vi "VSSNavigation.vi"(0 "output angle":dbl, 4 "output xy":dbl, 6 "Debug":bool, 8 "GoTo Navigation":bool, 11 "IA State Output in":T1) -> (3 "IA State Output out":T1)   [LabVIEW 2018]
uses:
  Vision_class/Old vision/SSL Detection Frame Simple Estimator Cameras VelCmd Folder/Core/AI Input.ctl
  Vision_class/Old vision/Controls/AI Robot.ctl
  Vision_class/Old vision/Controls/Functions Enum.ctl
  Vision_class/Old vision/Controls/AttackerStates.ctl
  Vision_class/Old vision/Controls/PathDests.ctl
  Vision_class/Old vision/Controls/PathDest.ctl
  VSSAttackerStates.ctl
  Vision_class/Old vision/SSL Detection Frame Simple Estimator Cameras VelCmd Folder/Core/AI Ball.ctl
  Vision_class/Old vision/SSL Detection Frame Simple Estimator Cameras VelCmd Folder/Core/Field Size.ctl
  Vision_class/Old vision/SSL Detection Frame Simple Estimator Cameras VelCmd Folder/Core/AI Judge.ctl
  Communication_class/Paths/MessageAI_State Folder/Intel/Command Enum.ctl
  Vision_class/Old vision/SSL Detection Frame Simple Estimator Cameras VelCmd Folder/Util/Events/Events.ctl
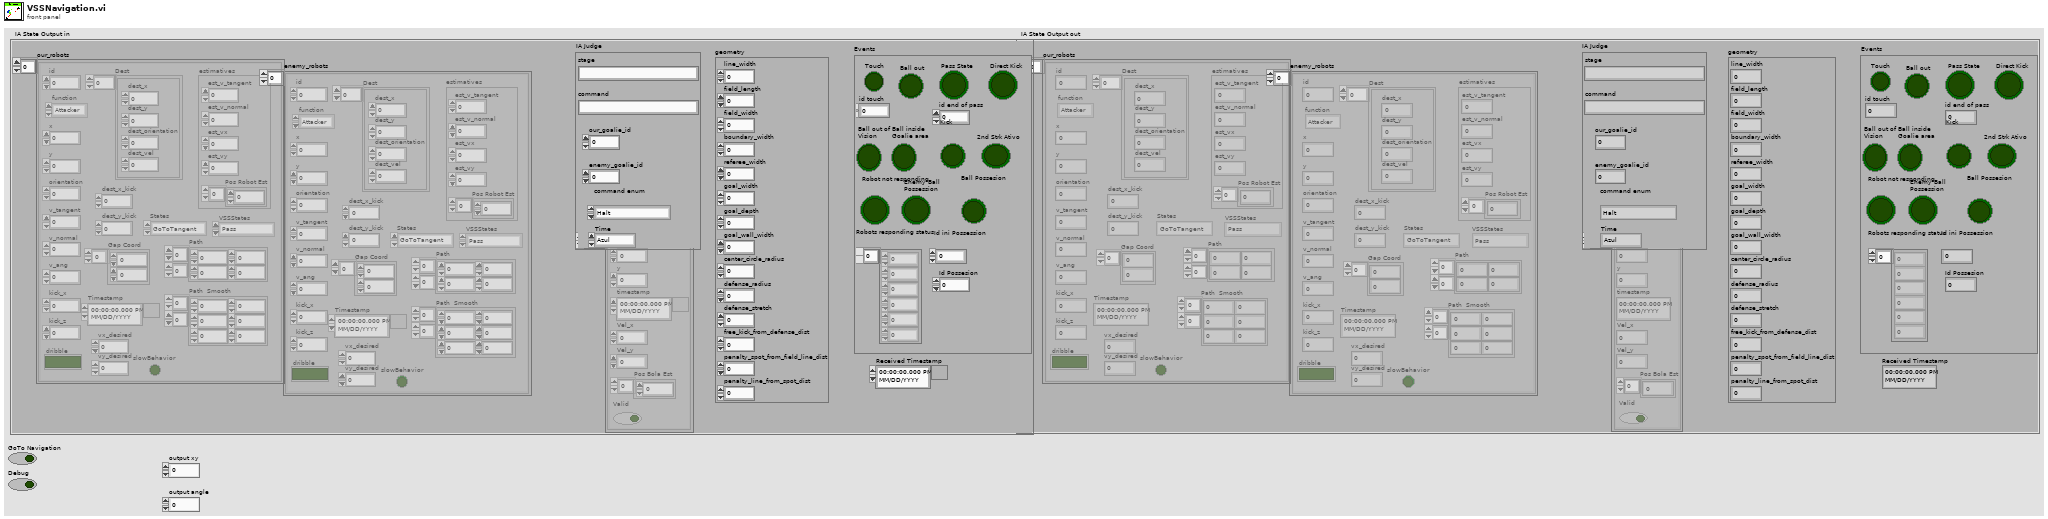
[diagram p1: front panel]
types:
  T1 = typedef "AI Input.ctl" = cluster{"our_robots":T2[], "enemy_robots":T2[], "balls":T8[], "geometry":T9, "IA Judge":T10, "Received Timestamp":timestamp, "Events":T12}
  T2 = typedef "AI Robot.ctl" = cluster{"id":u32, "function":T3, "x":dbl, "y":dbl, "orientation":dbl, "v_tangent":dbl, "v_normal":dbl, "v_ang":dbl, "kick_x":dbl, "kick_z":dbl, "dribble":bool, "Timestamp":timestamp, "estimatives":cluster{"est_v_tangent":dbl, "est_v_normal":dbl, "est_vx":dbl, "est_vy":dbl, "Pos Robot Est":dbl[]}, "dest_x_kick":dbl, "dest_y_kick":dbl, "Gap Coord":dbl[], "States":T4, "Path ":dbl[][], "Path  Smooth":dbl[][], "Dest":T5, "vx_desired":dbl, "vy_desired":dbl, "slowBehavior":bool, "VSSStates":T7}
  T3 = typedef "Functions Enum.ctl" = enum16{"2nd Striker", "Attacker", "Goalie", "Defender", "Striker", "Goto 0", "Dummy", "Kicker", "ZigZag 0", "ZigZag 1", "ZigZag 2", "ZigZag 3", "ZigZag 4", "ZigZag 5", "ZigZag 6", "ZigZag 7", "ZigZag 8", ""}
  T4 = typedef "AttackerStates.ctl" = enum16{"Pass", "GoToTangent", "BallGetting", "GoToKick", ""}
  T5 = typedef "PathDests.ctl" = T6[]
  T6 = typedef "PathDest.ctl" = cluster{"dest_x":dbl, "dest_y":dbl, "dest_orientation":dbl, "dest_vel":dbl}
  T7 = typedef "VSSAttackerStates.ctl" = enum16{"Pass", "GoToTangent", "BallGetting", "GoToKick", "Rotate anti-clockwise", "Rotate Clockwise", ""}
  T8 = typedef "AI Ball.ctl" = cluster{"x":dbl, "y":dbl, "timestamp":timestamp, "Vel_x":dbl, "Vel_y":dbl, "Pos Bola Est":dbl[], "Valid":bool}
  T9 = typedef "Field Size.ctl" = cluster{"line_width":u32, "field_length":u32, "field_width":u32, "boundary_width":u32, "referee_width":u32, "goal_width":u32, "goal_depth":u32, "goal_wall_width":u32, "center_circle_radius":u32, "defense_radius":u32, "defense_stretch":u32, "free_kick_from_defense_dist":u32, "penalty_spot_from_field_line_dist":u32, "penalty_line_from_spot_dist":u32}
  T10 = typedef "AI Judge.ctl" = cluster{"stage":string, "command":string, "our_goalie_id":dbl, "enemy_goalie_id":dbl, "command enum":T11, "Time":enum16{"Azul", "Amarelo"}}
  T11 = typedef "Command Enum.ctl" = enum16{"Halt", "Stop", "Force Start", "PKA Normal Start", "Prepare Kickoff Ally", "PKE Normal Start", "Prepare Kickoff Enemy", "Prepare Penalty Ally", "PPA Normal Start", "Prepare Penalty Enemy", "PPE Normal Start", "Direct Free Enemy", "Direct Free Ally", "Indirect Free Enemy", "Indirect Free Ally", "Timeout Enemy", "Timeout Ally", "Goal Enemy", "Goal Ally", "Ball Placement Enemy", "Ball Placement Ally", "Normal Half Time", "Extra Time Break", "Extra Half Time", "None", "Post Game"}
  T12 = typedef "Events.ctl" = cluster{"Touch":bool, "Ball out":bool, "id touch":dbl, "Ball out of \nVision":bool, "Ball inside \nGoalie area":bool, "Robot not responding":bool, "Robots responding status":dbl[], "Enemy Ball \nPossession":bool, "Pass State":bool, "id end of pass":dbl, "Kick":bool, "Id ini Possession":dbl, "Ball Possesion":bool, "Id Possesion":dbl, "Direct Kick":bool, "2nd Strk Ativo":bool}
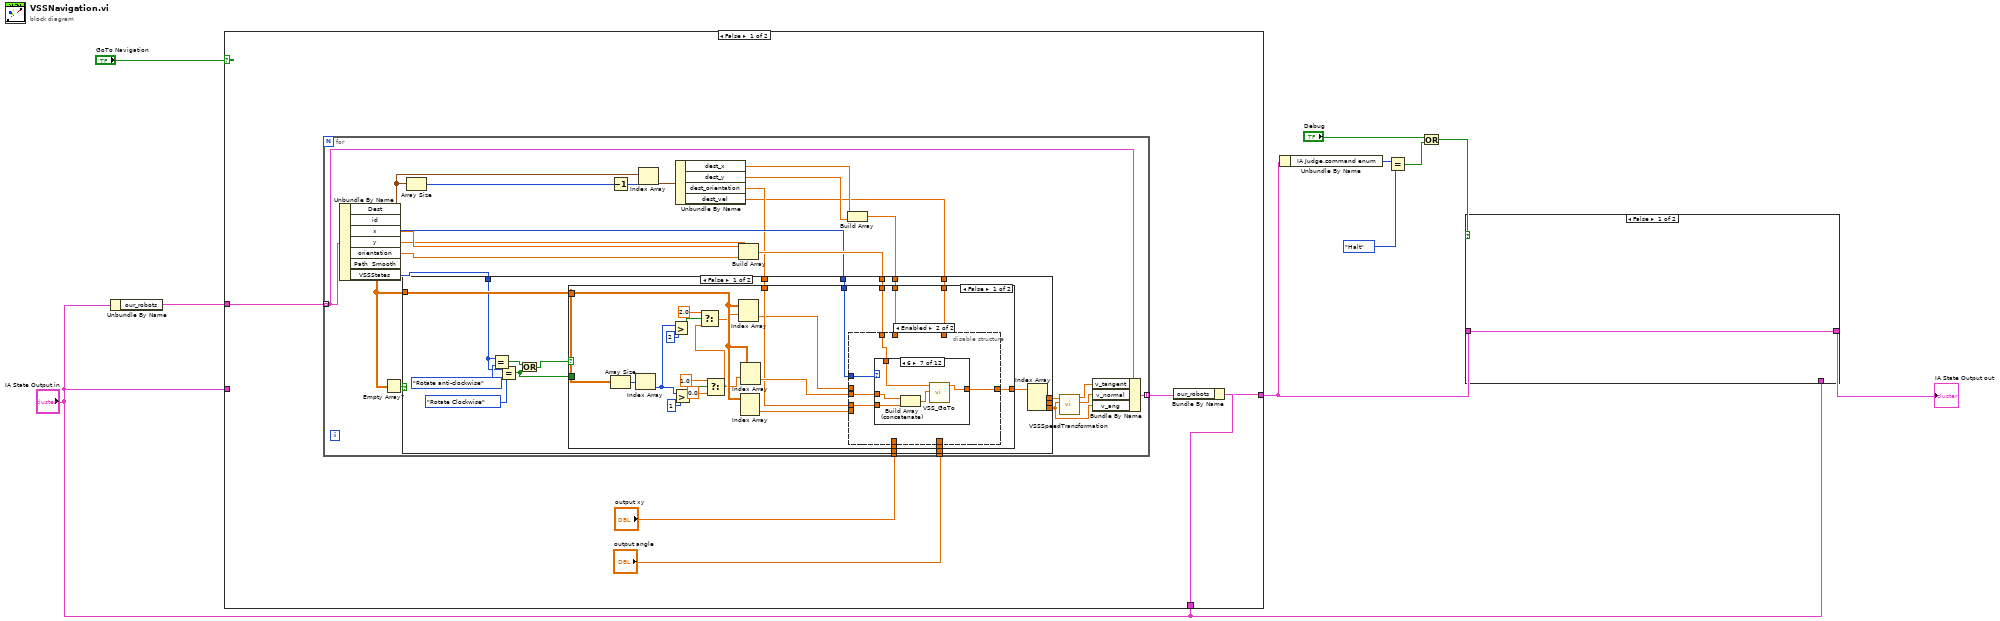
[diagram p0: block diagram]
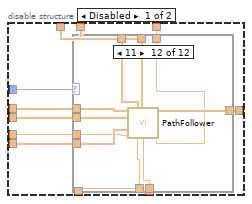
[diagram p2: hidden frame]
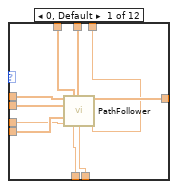
[diagram p3: hidden frame]
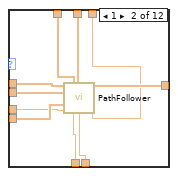
[diagram p4: hidden frame]
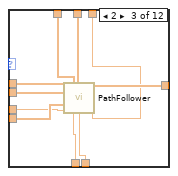
[diagram p5: hidden frame]
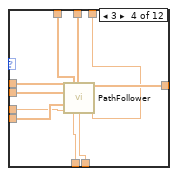
[diagram p6: hidden frame]
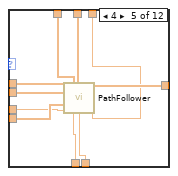
[diagram p7: hidden frame]
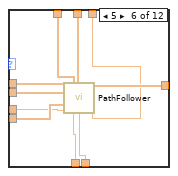
[diagram p8: hidden frame]
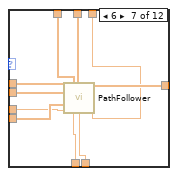
[diagram p9: hidden frame]
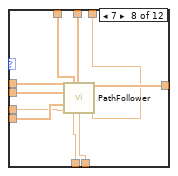
[diagram p10: hidden frame]
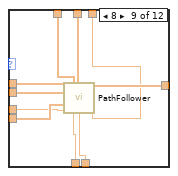
[diagram p11: hidden frame]
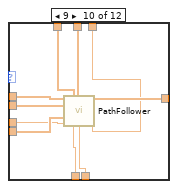
[diagram p12: hidden frame]
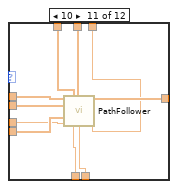
[diagram p13: hidden frame]
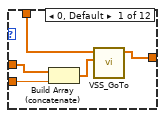
[diagram p14: hidden frame]
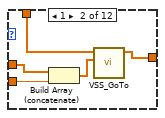
[diagram p15: hidden frame]
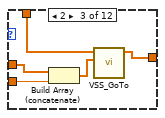
[diagram p16: hidden frame]
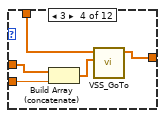
[diagram p17: hidden frame]
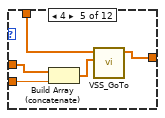
[diagram p18: hidden frame]
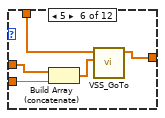
[diagram p19: hidden frame]
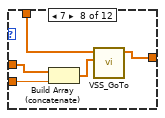
[diagram p20: hidden frame]
diagram:
  n1 = Unbundle By Name("IA State Output in") -> ("our_robots"=w10:T2[])
  n2 = case shown="False" "GoTo Navigation" {
    tunnel: w10 -> [w16 _]
    tunnel: [w13 w286] -> w6
    tunnel: "IA State Output in" -> [_ w287]
    tunnel: "IA State Output in" -> [w14 _]
    frame False {
      n3 = for {
        tunnel: w16 -> [w22] mode=indexing
        tunnel: [w37] -> w15 mode=indexing
        tunnel: "output xy" -> [w35]
        tunnel: "output angle" -> [w34]
        n4 = Unbundle By Name(w22) -> ("Dest"=w32:T5, "id"=w36:u32, "x"=w41:dbl, "y"=w40:dbl, "orientation"=w39:dbl, "Path  Smooth"=w23:dbl[][], "VSSStates"=w21:T7)
        n5 = Empty Array?(array=w23) -> (empty?=w24:bool)
        n6 = Array Size(array=w32) -> (size(s)=w31:i32)
        n7 = Decrement(x=w31) -> (x-1=w30:i32)
        n8 = Index Array(array=w32, index=w30) -> (element=w29:T6)
        n9 = Unbundle By Name(w29) -> ("dest_x"=w28:dbl, "dest_y"=w27:dbl, "dest_orientation"=w26:dbl, "dest_vel"=w25:dbl)
        n10 = Build Array(w41, w40, w39) -> (w38:dbl[])
        n11 = Build Array(w28, w27) -> (w33:dbl[])
        n12 = case shown="False" w24 {
          tunnel: w38 -> [w59 _]
          tunnel: [w57 w285] -> w20
          tunnel: [w56 w285] -> _
          tunnel: [w55 w285] -> w17
          tunnel: w36 -> [w54 _]
          tunnel: w35 -> [w53 _]
          tunnel: w34 -> [w52 _]
          tunnel: w23 -> [w48 _]
          tunnel: w33 -> [w51 _]
          tunnel: w26 -> [w50 _]
          tunnel: w25 -> [w49 _]
          tunnel: w21 -> [w45 _]
          frame False {
            n13 = Equal?(x=w45, y=VSSAttackerStates."Rotate anti-clockwise" ("States")) -> (x = y?=w44:bool)
            n14 = Equal?(x=w45, y=VSSAttackerStates."Rotate Clockwise" ("States")) -> (x = y?=w42:bool)
            n15 = Or(x=w44, y=w42) -> (x .or. y?=w43:bool)
            n16 = case shown="False" w43 {
              tunnel: w59 -> [w82 _]
              tunnel: [w81 w284] -> w58
              tunnel: w54 -> [w75 _]
              tunnel: w53 -> [w72 _]
              tunnel: w52 -> [w71 _]
              tunnel: w51 -> [w70 _]
              tunnel: w50 -> [w69 _]
              tunnel: w49 -> [w68 _]
              tunnel: w48 -> [w64 _]
              tunnel: w42 -> [_ w282]
              frame False {
                n17 = Array Size(array=w64) -> (size(s)=w80:i32[])
                n18 = Index Array(array=w80) -> (element=w61:i32)  [unwired: 1 in]
                n19 = Greater?(x=w61, y=2) -> (0:w65:bool)
                n20 = Greater?(x=w61, y=1) -> (0:w79:bool)
                n21 = Select(t=1.0, s=w79, f=0.0) -> (s? t:f=w62:dbl)
                n22 = Select(t=2.0, s=w65, f=w62) -> (s? t:f=w63:dbl)
                n23 = Index Array(array=w64, index (row)=w63) -> (element=w60:dbl[])  [unwired: 1 in]
                n24 = Index Array(array=w64) -> (element=w73:dbl[])  [unwired: 2 in]
                n25 = Index Array(array=w64, index (row)=w62) -> (element=w74:dbl[])  [unwired: 1 in]
                n26 = disable-structure shown="Enabled" {
                  disable-tunnel: w82 -> [w93 w216]
                  disable-tunnel: [w92 w215] -> w81
                  disable-tunnel: w75 -> [w91 w218]
                  disable-tunnel: w74 -> [w90 w217]
                  disable-tunnel: w73 -> [w89 _]
                  disable-tunnel: w72 -> [w88 _]
                  disable-tunnel: w71 -> [w87 _]
                  disable-tunnel: w70 -> [w86 _]
                  disable-tunnel: w69 -> [w85 w214]
                  disable-tunnel: w68 -> [w84 _]
                  disable-tunnel: w60 -> [w83 _]
                  frame Disabled {
                    n27 = case shown="11" w91 {
                      tunnel: w90 -> [w102 w112 w122 w132 w142 w152 w162 w172 w182 w192 w202 w212]
                      tunnel: w93 -> [w98 w108 w118 w128 w138 w148 w158 w168 w178 w188 w198 w208]
                      tunnel: [w103 w113 w123 w133 w143 w153 w163 w173 w183 w193 w203 w213] -> w92
                      tunnel: w89 -> [w101 w111 w121 w131 w141 w151 w161 w171 w181 w191 w201 w211]
                      tunnel: w88 -> [w100 w110 w120 w130 w140 w150 w160 w170 w180 w190 w200 w210]
                      tunnel: w87 -> [w99 w109 w119 w129 w139 w149 w159 w169 w179 w189 w199 w209]
                      tunnel: w86 -> [w97 w107 w117 w127 w137 w147 w157 w167 w177 w187 w197 w207]
                      tunnel: w85 -> [w96 w106 w116 w126 w136 w146 w156 w166 w176 w186 w196 w206]
                      tunnel: w84 -> [w95 w105 w115 w125 w135 w145 w155 w165 w175 w185 w195 w205]
                      tunnel: w83 -> [w94 w104 w114 w124 w134 w144 w154 w164 w174 w184 w194 w204]
                      frame 0, Default {
                        n28 = call "PathFollower.vi"("Waypoint 2"=w94, "Position"=w98, "Dest"=w97, "Waypoint 1"=w102, "Waypoint 0"=w101, "Dest_orientation"=w96, "output xy"=w100, "output angle"=w99, "dest_vel"=w95) -> ("Output\nVelocity"=w103:dbl[])  [unwired: 6 in]
                      }
                      frame 1 {
                        n29 = call "PathFollower.vi"("Waypoint 2"=w104, "Position"=w108, "Dest"=w107, "Waypoint 1"=w112, "Waypoint 0"=w111, "Dest_orientation"=w106, "output xy"=w110, "output angle"=w109, "dest_vel"=w105) -> ("Output\nVelocity"=w113:dbl[])  [unwired: 6 in]
                      }
                      frame 2 {
                        n30 = call "PathFollower.vi"("Waypoint 2"=w114, "Position"=w118, "Dest"=w117, "Waypoint 1"=w122, "Waypoint 0"=w121, "Dest_orientation"=w116, "output xy"=w120, "output angle"=w119, "dest_vel"=w115) -> ("Output\nVelocity"=w123:dbl[])  [unwired: 6 in]
                      }
                      frame 3 {
                        n31 = call "PathFollower.vi"("Waypoint 2"=w124, "Position"=w128, "Dest"=w127, "Waypoint 1"=w132, "Waypoint 0"=w131, "Dest_orientation"=w126, "output xy"=w130, "output angle"=w129, "dest_vel"=w125) -> ("Output\nVelocity"=w133:dbl[])  [unwired: 6 in]
                      }
                      frame 4 {
                        n32 = call "PathFollower.vi"("Waypoint 2"=w134, "Position"=w138, "Dest"=w137, "Waypoint 1"=w142, "Waypoint 0"=w141, "Dest_orientation"=w136, "output xy"=w140, "output angle"=w139, "dest_vel"=w135) -> ("Output\nVelocity"=w143:dbl[])  [unwired: 6 in]
                      }
                      frame 5 {
                        n33 = call "PathFollower.vi"("Waypoint 2"=w144, "Position"=w148, "Dest"=w147, "Waypoint 1"=w152, "Waypoint 0"=w151, "Dest_orientation"=w146, "output xy"=w150, "output angle"=w149, "dest_vel"=w145) -> ("Output\nVelocity"=w153:dbl[])  [unwired: 6 in]
                      }
                      frame 6 {
                        n34 = call "PathFollower.vi"("Waypoint 2"=w154, "Position"=w158, "Dest"=w157, "Waypoint 1"=w162, "Waypoint 0"=w161, "Dest_orientation"=w156, "output xy"=w160, "output angle"=w159, "dest_vel"=w155) -> ("Output\nVelocity"=w163:dbl[])  [unwired: 6 in]
                      }
                      frame 7 {
                        n35 = call "PathFollower.vi"("Waypoint 2"=w164, "Position"=w168, "Dest"=w167, "Waypoint 1"=w172, "Waypoint 0"=w171, "Dest_orientation"=w166, "output xy"=w170, "output angle"=w169, "dest_vel"=w165) -> ("Output\nVelocity"=w173:dbl[])  [unwired: 6 in]
                      }
                      frame 8 {
                        n36 = call "PathFollower.vi"("Waypoint 2"=w174, "Position"=w178, "Dest"=w177, "Waypoint 1"=w182, "Waypoint 0"=w181, "Dest_orientation"=w176, "output xy"=w180, "output angle"=w179, "dest_vel"=w175) -> ("Output\nVelocity"=w183:dbl[])  [unwired: 6 in]
                      }
                      frame 9 {
                        n37 = call "PathFollower.vi"("Waypoint 2"=w184, "Position"=w188, "Dest"=w187, "Waypoint 1"=w192, "Waypoint 0"=w191, "Dest_orientation"=w186, "output xy"=w190, "output angle"=w189, "dest_vel"=w185) -> ("Output\nVelocity"=w193:dbl[])  [unwired: 6 in]
                      }
                      frame 10 {
                        n38 = call "PathFollower.vi"("Waypoint 2"=w194, "Position"=w198, "Dest"=w197, "Waypoint 1"=w202, "Waypoint 0"=w201, "Dest_orientation"=w196, "output xy"=w200, "output angle"=w199, "dest_vel"=w195) -> ("Output\nVelocity"=w203:dbl[])  [unwired: 6 in]
                      }
                      frame 11 {
                        n39 = call "PathFollower.vi"("Waypoint 2"=w204, "Position"=w208, "Dest"=w207, "Waypoint 1"=w212, "Waypoint 0"=w211, "Dest_orientation"=w206, "output xy"=w210, "output angle"=w209, "dest_vel"=w205) -> ("Output\nVelocity"=w213:dbl[])  [unwired: 6 in]
                      }
                    }
                  }
                  frame Enabled {
                    n40 = case shown="6" w218 {
                      tunnel: w217 -> [w221 w226 w231 w236 w241 w246 w251 w256 w261 w266 w271 w276]
                      tunnel: w216 -> [w223 w228 w233 w238 w243 w248 w253 w258 w263 w268 w273 w278]
                      tunnel: [w222 w227 w232 w237 w242 w247 w252 w257 w262 w267 w272 w277] -> w215
                      tunnel: w214 -> [w220 w225 w230 w235 w240 w245 w250 w255 w260 w265 w270 w275]
                      frame 0, Default {
                        n41 = Build Array (concatenate)(w221, w220) -> (w219:dbl[])
                        n42 = call "VSS_GoTo.vi"("SetPoint"=w219, "Position"=w223) -> ("Output Vel"=w222:dbl[])  [unwired: 9 in]
                      }
                      frame 1 {
                        n43 = Build Array (concatenate)(w226, w225) -> (w224:dbl[])
                        n44 = call "VSS_GoTo.vi"("SetPoint"=w224, "Position"=w228) -> ("Output Vel"=w227:dbl[])  [unwired: 9 in]
                      }
                      frame 2 {
                        n45 = Build Array (concatenate)(w231, w230) -> (w229:dbl[])
                        n46 = call "VSS_GoTo.vi"("SetPoint"=w229, "Position"=w233) -> ("Output Vel"=w232:dbl[])  [unwired: 9 in]
                      }
                      frame 3 {
                        n47 = Build Array (concatenate)(w236, w235) -> (w234:dbl[])
                        n48 = call "VSS_GoTo.vi"("SetPoint"=w234, "Position"=w238) -> ("Output Vel"=w237:dbl[])  [unwired: 9 in]
                      }
                      frame 4 {
                        n49 = Build Array (concatenate)(w241, w240) -> (w239:dbl[])
                        n50 = call "VSS_GoTo.vi"("SetPoint"=w239, "Position"=w243) -> ("Output Vel"=w242:dbl[])  [unwired: 9 in]
                      }
                      frame 5 {
                        n51 = Build Array (concatenate)(w246, w245) -> (w244:dbl[])
                        n52 = call "VSS_GoTo.vi"("SetPoint"=w244, "Position"=w248) -> ("Output Vel"=w247:dbl[])  [unwired: 9 in]
                      }
                      frame 6 {
                        n53 = Build Array (concatenate)(w251, w250) -> (w249:dbl[])
                        n54 = call "VSS_GoTo.vi"("SetPoint"=w249, "Position"=w253) -> ("Output Vel"=w252:dbl[])  [unwired: 9 in]
                      }
                      frame 7 {
                        n55 = Build Array (concatenate)(w256, w255) -> (w254:dbl[])
                        n56 = call "VSS_GoTo.vi"("SetPoint"=w254, "Position"=w258) -> ("Output Vel"=w257:dbl[])  [unwired: 9 in]
                      }
                      frame 8 {
                        n57 = Build Array (concatenate)(w261, w260) -> (w259:dbl[])
                        n58 = call "VSS_GoTo.vi"("SetPoint"=w259, "Position"=w263) -> ("Output Vel"=w262:dbl[])  [unwired: 9 in]
                      }
                      frame 9 {
                        n59 = Build Array (concatenate)(w266, w265) -> (w264:dbl[])
                        n60 = call "VSS_GoTo.vi"("SetPoint"=w264, "Position"=w268) -> ("Output Vel"=w267:dbl[])  [unwired: 9 in]
                      }
                      frame 10 {
                        n61 = Build Array (concatenate)(w271, w270) -> (w269:dbl[])
                        n62 = call "VSS_GoTo.vi"("SetPoint"=w269, "Position"=w273) -> ("Output Vel"=w272:dbl[])  [unwired: 9 in]
                      }
                      frame 11 {
                        n63 = Build Array (concatenate)(w276, w275) -> (w274:dbl[])
                        n64 = call "VSS_GoTo.vi"("SetPoint"=w274, "Position"=w278) -> ("Output Vel"=w277:dbl[])  [unwired: 9 in]
                      }
                    }
                  }
                }
              }
              frame True {
                w280 = 3.0 ("element")
                w283 = 0.0 ("element")
                n65 = Negate(x=w280) -> (-x=w281:dbl)
                n66 = Select(t=w280, s=w282, f=w281) -> (s? t:f=w279:dbl)
                n67 = Build Array(w283, w283, w279) -> (w284:dbl[])
              }
            }
            n68 = Index Array(array=w58) -> (element #1=w57:dbl, element #2=w56:dbl, element #3=w55:dbl)  [unwired: 3 in]
          }
          frame True {
            w285 = 0.0 ("output")
          }
        }
        n69 = call "VSSSpeedTransformation.vi"("V_ang in"=w17, "V_tang in"=w20) -> ("V_rigth"=w18:dbl, "V_left"=w19:dbl)  [unwired: 8 in]
        n70 = Bundle By Name(cluster=w22, "v_tangent"=w19, "v_normal"=w18, "v_ang"=w17) -> (w37:T2)
      }
      n71 = Bundle By Name(cluster=w14, "our_robots"=w15) -> (w13:T1)
    }
    frame True {
      n72 = call "potential-field.vi"("IA State Output in"=w287) -> ("IA State Output out"=w286:T1)  [unwired: 10 in]
    }
  }
  n73 = Unbundle By Name(w6) -> ("IA Judge.command enum"=w5:T11)
  n74 = Equal?(x=w5, y=Command_Enum."Halt") -> (x = y?=w2:bool)
  n75 = Or(x="Debug", y=w2) -> (x .or. y?=w3:bool)
  n76 = case shown="False" w3 {
    tunnel: [w288 w293] -> w8
    tunnel: w6 -> [w288 w290]
    tunnel: "IA State Output in" -> [_ w291]
    frame False {
    }
    frame True {
      n77 = Unbundle By Name(w290) -> ("our_robots"=w289:T2[])
      n78 = for {
        tunnel: [w296] -> w292 mode=indexing
        tunnel: w289 -> [w294] mode=indexing
        w295 = 0.0 ("v_normal")
        n79 = Bundle By Name(cluster=w294, "v_tangent"=w295, "v_normal"=w295, "v_ang"=w295) -> (w296:T2)
      }
      n80 = Bundle By Name(cluster=w291, "our_robots"=w292) -> (w293:T1)
    }
  }
  "IA State Output out" <- w8
